vi "Flatten Pixmap 32-bit pixmap.vi"(4 "mask":u8[](array[numeric]), 5 "top left":cluster{"x":i16, "y":i16}, 6 "colors":u32[](array[numeric]), 7 "32-bit pixmap":u32[][](array[numeric]), 8 "1-bit pixmap":bool[][](array[boolean]), 9 "4-bit pixmap":u8[][](array[numeric]), 10 "8-bit pixmap":u8[][](array[numeric]), 11 "24-bit pixmap":u32[][](array[numeric])) -> (2 "image data":T1)   [LabVIEW 2021, in "Picture2D.lvlib"]
doc: "Converts pixmap data from a 2D array to a 1D array."
uses:
  Picture2D/Picture2D.lvlib
  <vilib>/picture/picture.llb/imagedata.ctl
panel:
  in  "image data":T1
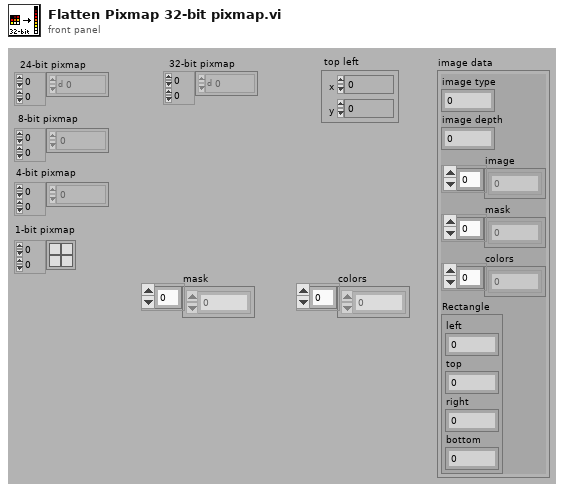
[diagram p1: front panel]
types:
  T1 = typedef "imagedata.ctl" = cluster{"image type":i32, "image depth":i32, "image":u8[], "mask":u8[], "colors":u32[], "Rectangle":cluster{"left":i16, "top":i16, "right":i16, "bottom":i16}}
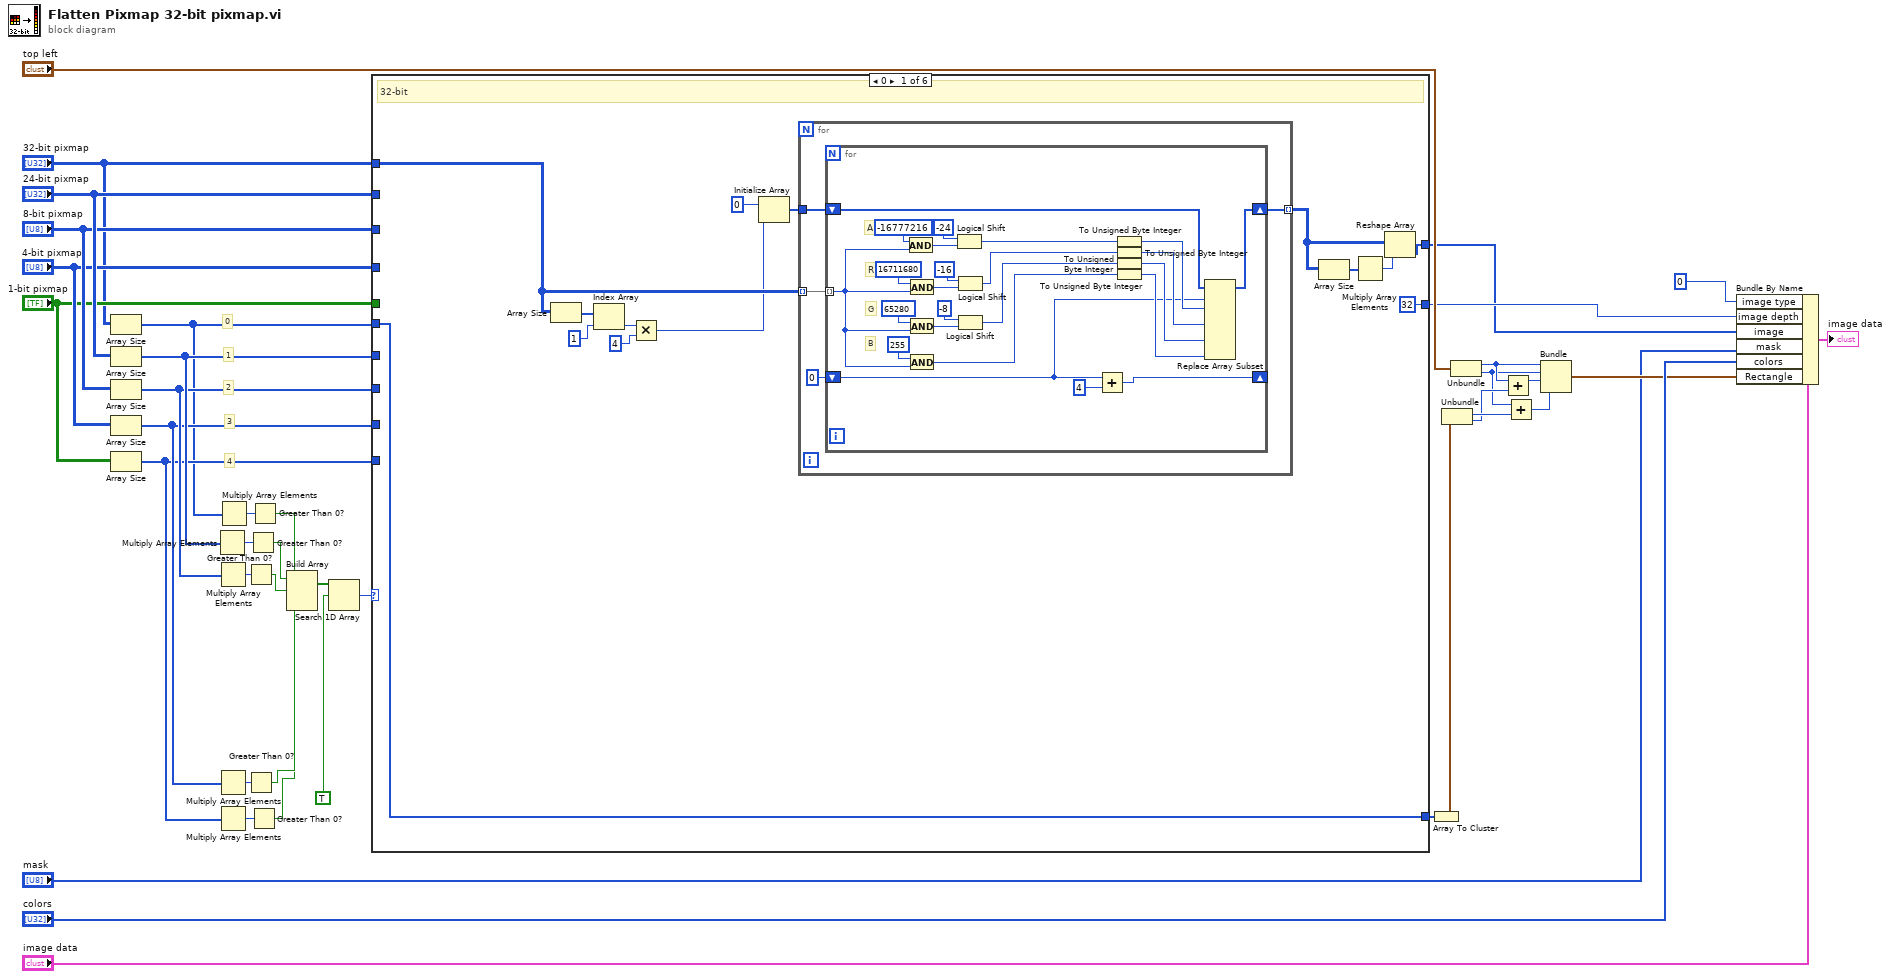
[diagram p0: block diagram]
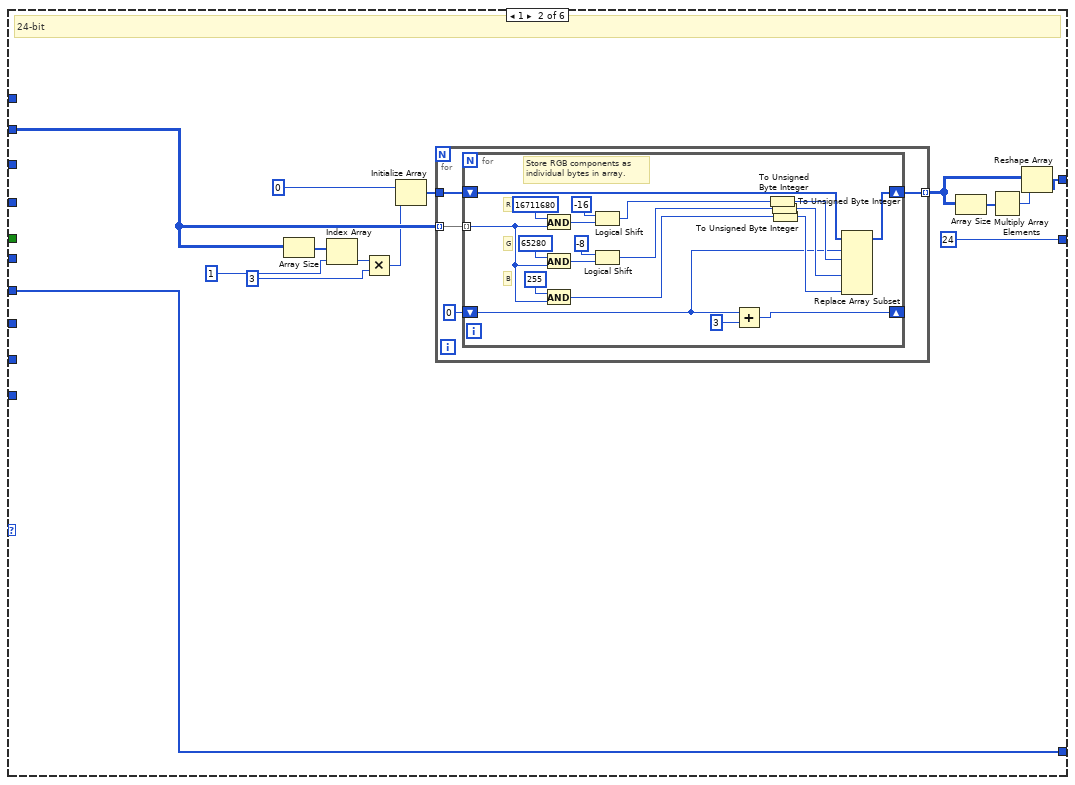
[diagram p2: hidden frame]
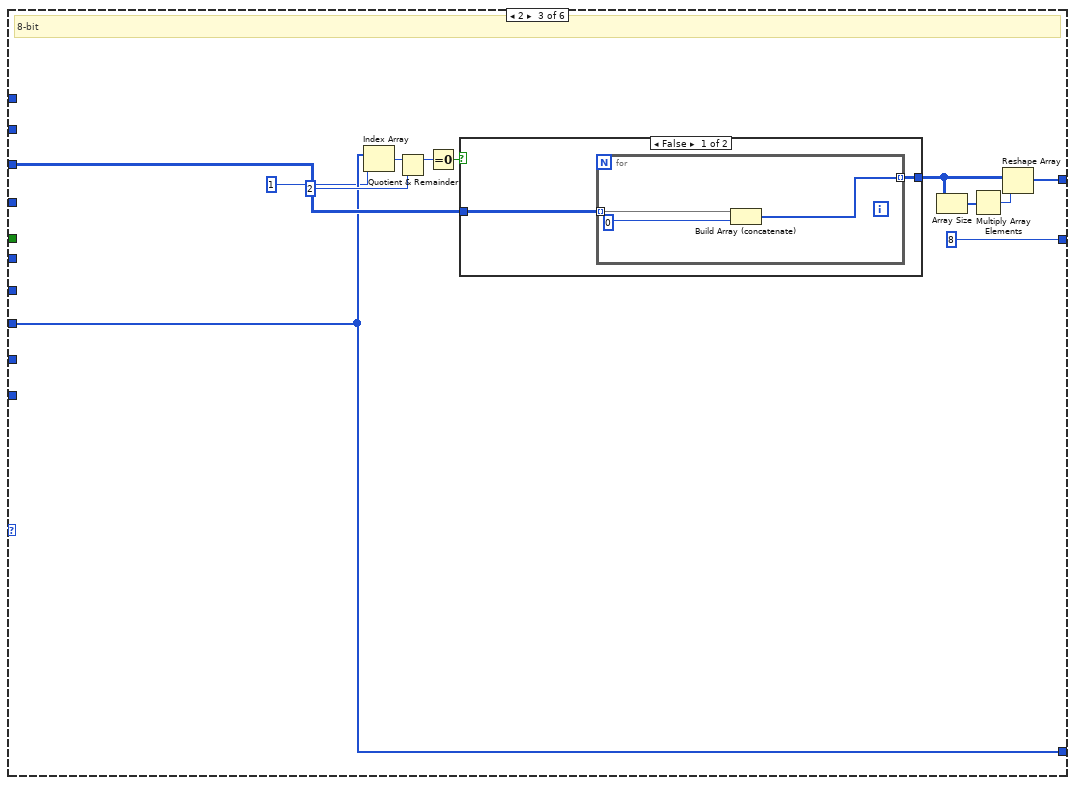
[diagram p3: hidden frame]
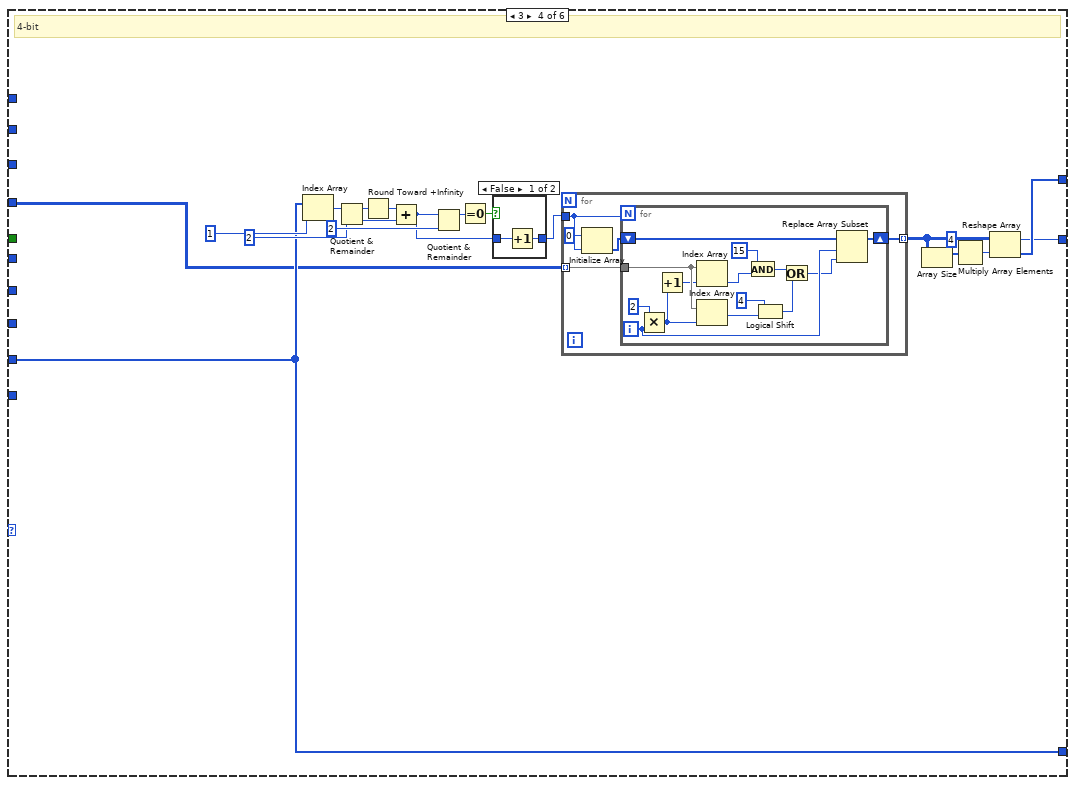
[diagram p5: hidden frame]
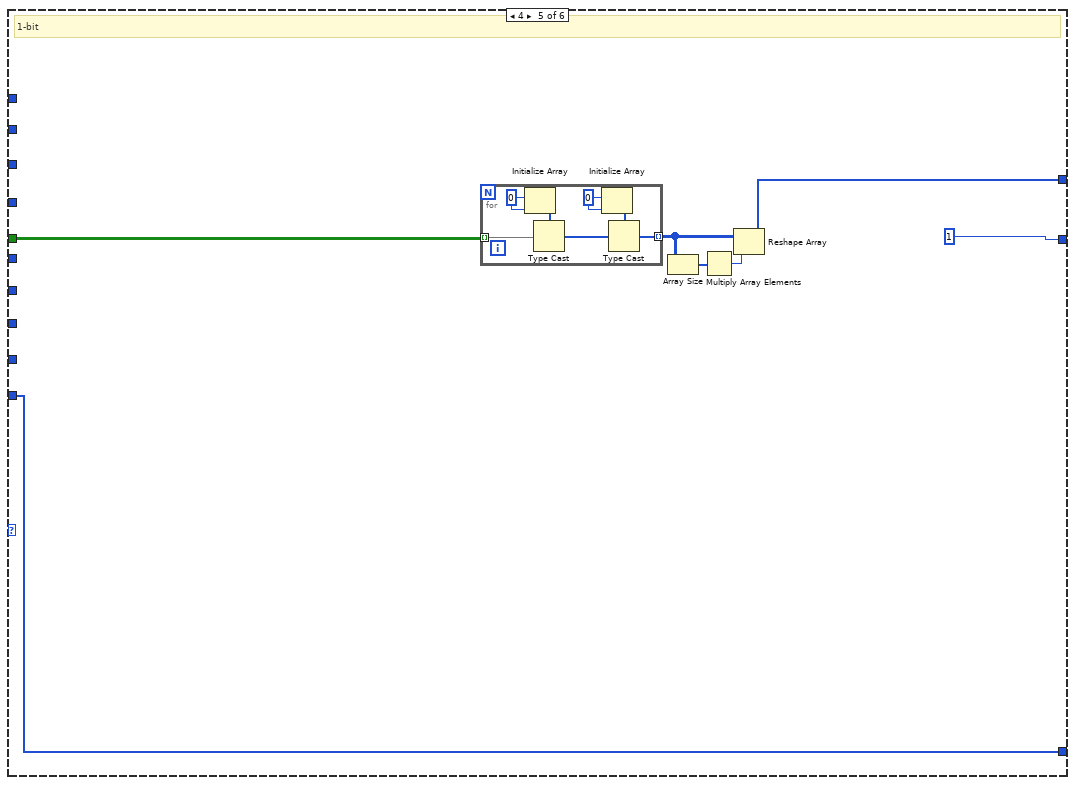
[diagram p7: hidden frame]
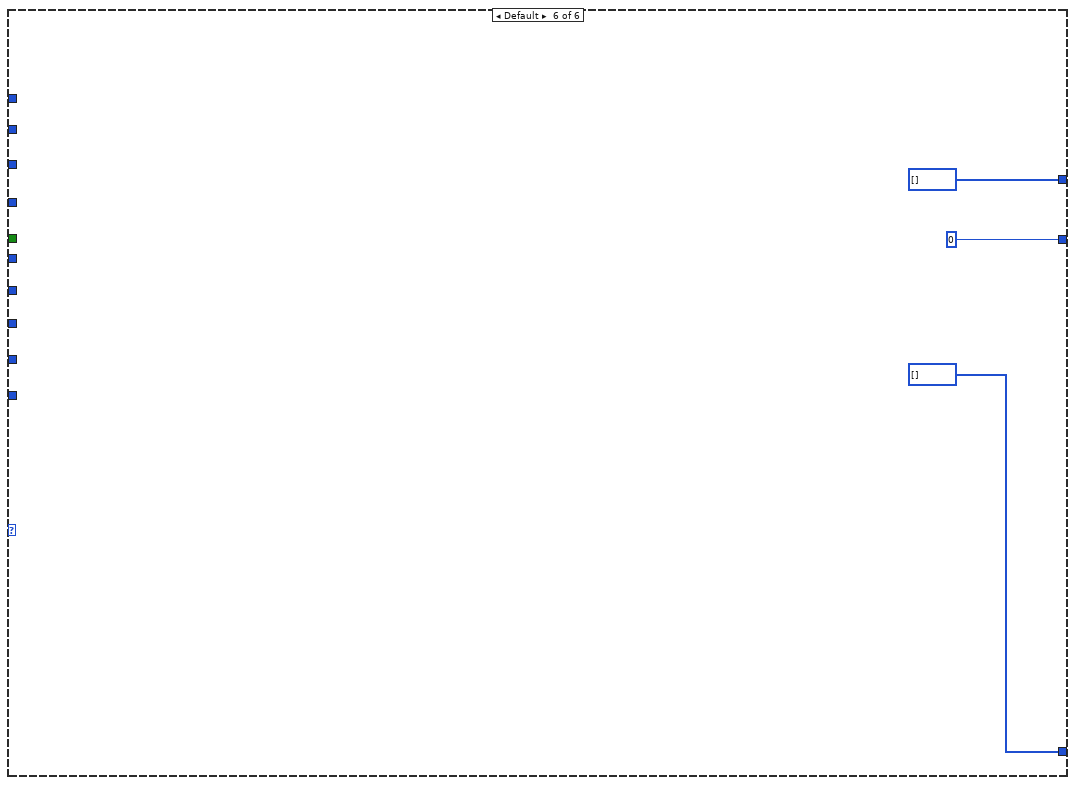
[diagram p8: hidden frame]
diagram:
  # "4"
  # "3"
  # "2"
  # "1"
  # "0"
  n1 = Array Size(array="32-bit pixmap") -> (size(s)=w1:i32[])
  n2 = Array Size(array="24-bit pixmap") -> (size(s)=w25:i32[])
  n3 = Array Size(array="8-bit pixmap") -> (size(s)=w24:i32[])
  n4 = Array Size(array="4-bit pixmap") -> (size(s)=w23:i32[])
  n5 = Array Size(array="1-bit pixmap") -> (size(s)=w22:i32[])
  n6 = Multiply Array Elements(1:w25) -> (0:w40:i32)
  n7 = Multiply Array Elements(1:w24) -> (0:w39:i32)
  n8 = Multiply Array Elements(1:w23) -> (0:w38:i32)
  n9 = Multiply Array Elements(1:w22) -> (0:w37:i32)
  n10 = Multiply Array Elements(1:w1) -> (0:w4:i32)
  n11 = Greater Than 0?(x=w39) -> (x > 0?=w34:bool)
  n12 = Greater Than 0?(x=w38) -> (x > 0?=w33:bool)
  n13 = Greater Than 0?(x=w40) -> (x > 0?=w35:bool)
  n14 = Greater Than 0?(x=w37) -> (x > 0?=w32:bool)
  n15 = Greater Than 0?(x=w4) -> (x > 0?=w2:bool)
  n16 = Build Array(w2, w35, w34, w33, w32) -> (w36:bool[])
  n17 = Search 1D Array(1D array=w36, element=TRUE) -> (index of element=w30:i32)  [unwired: 1 in]
  n18 = case shown="0" w30 {
    tunnel: [w54 w93 w126 w142 w180 u8[] [] ("8-bit pixmap")] -> w6
    tunnel: "24-bit pixmap" -> [_ w90 _ _ _ _]
    tunnel: "8-bit pixmap" -> [_ _ w125 _ _ _]
    tunnel: "4-bit pixmap" -> [_ _ _ w138 _ _]
    tunnel: "1-bit pixmap" -> [_ _ _ _ w181 _]
    tunnel: [32 24 8 4 1 0] -> w10
    tunnel: w25 -> [_ w91 _ _ _ _]
    tunnel: w24 -> [_ _ w122 _ _ _]
    tunnel: w23 -> [_ _ _ w140 _ _]
    tunnel: w22 -> [_ _ _ _ w178 _]
    tunnel: [w51 w91 w122 w140 w178 i32[] []] -> w21
    tunnel: "32-bit pixmap" -> [w52 _ _ _ _ _]
    tunnel: w1 -> [w51 _ _ _ _ _]
    frame 0 {
      # "32-bit"
      n19 = Array Size(array=w52) -> (size(s)=w47:i32[])
      n20 = Index Array(array=w47, index=1) -> (element=w45:i32)
      n21 = Multiply(x=w45, y=4) -> (x*y=w43:i32)
      n22 = Initialize Array(u8 0, w43) -> (w41:u8[])
      n23 = for {
        tunnel: w52 -> [w56] mode=indexing
        tunnel: [w58] -> w48 mode=indexing
        tunnel: w41 -> [w55]
        n24 = for {
          tunnel: w56 -> [w59] mode=indexing
          shift-right: [w67] -> w58
          shift-left: w55 -> [w68]
          shift-right: [w66] -> _
          shift-left: 0 -> [w60]
          # "A"
          # "B"
          # "G"
          # "R"
          n25 = And(x=-16777216, y=w59) -> (x .and. y?=w63:u32)
          n26 = And(x=16711680, y=w59) -> (x .and. y?=w77:u32)
          n27 = And(x=65280, y=w59) -> (x .and. y?=w76:u32)
          n28 = And(x=255, y=w59) -> (x .and. y?=w73:u32)
          n29 = Logical Shift(y=i8 -24, x=w63) -> (x << y=w62:u32)
          n30 = Logical Shift(y=i8 -16, x=w77) -> (x << y=w75:u32)
          n31 = Logical Shift(y=i8 -8, x=w76) -> (x << y=w74:u32)
          n32 = Add(x=w60, y=4) -> (x+y=w66:i32)
          n33 = To Unsigned Byte Integer(number=w62) -> (unsigned 8bit integer=w61:u8)
          n34 = To Unsigned Byte Integer(number=w75) -> (unsigned 8bit integer=w71:u8)
          n35 = To Unsigned Byte Integer(number=w74) -> (unsigned 8bit integer=w70:u8)
          n36 = To Unsigned Byte Integer(number=w73) -> (unsigned 8bit integer=w69:u8)
          n37 = Replace Array Subset(array=w68, new element #1=w61, index #1=w60, new element #2=w71, new element #3=w70, new element #4=w69) -> (w67:u8[])  [unwired: 3 in]
        }
      }
      n38 = Array Size(array=w48) -> (size(s)=w49:i32[])
      n39 = Multiply Array Elements(1:w49) -> (0:w50:i32)
      n40 = Reshape Array(w48, w50) -> (w54:u8[])
    }
    frame 1 {
      # "24-bit"
      n41 = Array Size(array=w90) -> (size(s)=w89:i32[])
      n42 = Index Array(array=w89, index=1) -> (element=w87:i32)
      n43 = Multiply(x=w87, y=3) -> (x*y=w85:i32)
      n44 = Initialize Array(u8 0, w85) -> (w83:u8[])
      n45 = for {
        tunnel: w90 -> [w98] mode=indexing
        tunnel: [w100] -> w94 mode=indexing
        tunnel: w83 -> [w97]
        n46 = for {
          tunnel: w98 -> [w109] mode=indexing
          shift-right: [w103] -> w100
          shift-left: w97 -> [w104]
          shift-right: [w102] -> _
          shift-left: 0 -> [w101]
          # "B"
          # "G"
          # "R"
          # "Store RGB components as\nindividual bytes in array."
          n47 = And(x=16711680, y=w109) -> (x .and. y?=w114:u32)
          n48 = And(x=65280, y=w109) -> (x .and. y?=w113:u32)
          n49 = And(x=255, y=w109) -> (x .and. y?=w110:u32)
          n50 = Logical Shift(y=i8 -16, x=w114) -> (x << y=w112:u32)
          n51 = Logical Shift(y=i8 -8, x=w113) -> (x << y=w111:u32)
          n52 = Add(x=w101, y=3) -> (x+y=w102:i32)
          n53 = To Unsigned Byte Integer(number=w112) -> (unsigned 8bit integer=w107:u8)
          n54 = To Unsigned Byte Integer(number=w111) -> (unsigned 8bit integer=w106:u8)
          n55 = To Unsigned Byte Integer(number=w110) -> (unsigned 8bit integer=w105:u8)
          n56 = Replace Array Subset(array=w104, new element #1=w107, index #1=w101, new element #2=w106, new element #3=w105) -> (w103:u8[])  [unwired: 2 in]
        }
      }
      n57 = Array Size(array=w94) -> (size(s)=w95:i32[])
      n58 = Multiply Array Elements(1:w95) -> (0:w96:i32)
      n59 = Reshape Array(w94, w96) -> (w93:u8[])
    }
    frame 2 {
      # "8-bit"
      n60 = Index Array(array=w122, index=1) -> (element=w121:i32)
      n61 = Quotient & Remainder(x=w121, y=2) -> (x-y*floor(x/y)=w127:i32)  [unwired: 1 out]
      n62 = Equal To 0?(x=w127) -> (x = 0?=w124:bool)
      n63 = case shown="False" w124 {
        tunnel: [w132 w137] -> w129
        tunnel: w125 -> [w133 w137]
        frame False {
          n64 = for {
            tunnel: w133 -> [w136] mode=indexing
            tunnel: [w134] -> w132 mode=indexing
            n65 = Build Array (concatenate)(w136, u8 0) -> (w134:u8[])
          }
        }
        frame True {
        }
      }
      n66 = Array Size(array=w129) -> (size(s)=w130:i32[])
      n67 = Multiply Array Elements(1:w130) -> (0:w131:i32)
      n68 = Reshape Array(w129, w131) -> (w126:u8[])
    }
    frame 3 {
      # "4-bit"
      n69 = Index Array(array=w140, index=1) -> (element=w154:i32)
      n70 = Quotient & Remainder(x=w154, y=2) -> (x-y*floor(x/y)=w148:i32, floor(x/y)=w146:i32)
      n71 = Round Toward +Infinity(x=w148) -> (ceil(x): smallest int >= x=w147:i32)
      n72 = Add(x=w147, y=w146) -> (x+y=w145:i32)
      n73 = Quotient & Remainder(x=w145, y=2) -> (x-y*floor(x/y)=w151:i32)  [unwired: 1 out]
      n74 = Equal To 0?(x=w151) -> (x = 0?=w150:bool)
      n75 = case shown="False" w150 {
        tunnel: w145 -> [w157 w158]
        tunnel: [w156 w158] -> w139
        frame False {
          n76 = Increment(x=w157) -> (x+1=w156:i32)
        }
        frame True {
        }
      }
      n77 = for {
        tunnel: w138 -> [w163] mode=indexing
        tunnel: [w162] -> w144 mode=indexing
        tunnel: w139 -> [w160]
        n78 = Initialize Array(u8 0, w160) -> (w159:u8[])
        n79 = for {
          N: w160 -> [_]
          tunnel: w163 -> [w177]
          shift-right: [w167] -> w162
          shift-left: w159 -> [w164]
          i -> [w166]
          n80 = Multiply(x=2, y=w166) -> (x*y=w175:i32)
          n81 = Increment(x=w175) -> (x+1=w174:i32)
          n82 = Index Array(array=w177, index=w174) -> (element=w173:u8)
          n83 = Index Array(array=w177, index=w175) -> (element=w171:u8)
          n84 = And(x=u8 15, y=w173) -> (x .and. y?=w170:u8)
          n85 = Logical Shift(y=u8 4, x=w171) -> (x << y=w169:u8)
          n86 = Or(x=w170, y=w169) -> (x .or. y?=w165:u8)
          n87 = Replace Array Subset(array=w164, new element=w165, index=w166) -> (w167:u8[])
        }
      }
      n88 = Array Size(array=w144) -> (size(s)=w143:i32[])
      n89 = Multiply Array Elements(1:w143) -> (0:w152:i32)
      n90 = Reshape Array(w144, w152) -> (w142:u8[])
    }
    frame 4 {
      # "1-bit"
      n91 = for {
        tunnel: [w188] -> w184 mode=indexing
        tunnel: w181 -> [w185] mode=indexing
        w187 = u8 0
        w190 = i16 0
        n92 = Initialize Array(w190, w190) -> (w191:i16[])
        n93 = Type Cast(type=w191, x=w185) -> (*(type *) &x=w189:i16[])
        n94 = Initialize Array(w187, w187) -> (w186:u8[])
        n95 = Type Cast(type=w186, x=w189) -> (*(type *) &x=w188:u8[])
      }
      n96 = Array Size(array=w184) -> (size(s)=w182:i32[])
      n97 = Multiply Array Elements(1:w182) -> (0:w183:i32)
      n98 = Reshape Array(w184, w183) -> (w180:u8[])
    }
    frame Default {
    }
  }
  n99 = Array To Cluster(array=w21) -> (cluster=w20:cluster{"[0]":i32, "[1]":i32})
  n100 = Unbundle(w20) -> ("[0]"=w19:i32, "[1]"=w16:i32)
  n101 = Unbundle("top left") -> ("x"=w17:i16, "y"=w15:i16)
  n102 = Add(x=w17, y=w16) -> (x+y=w13:i32)
  n103 = Add(x=w15, y=w19) -> (x+y=w14:i32)
  n104 = Bundle("x"=w17, "y"=w15, w13, w14) -> (w8:cluster{"x":i16, "y":i16, i32, i32})  [unwired: 1 in]
  n105 = Bundle By Name(cluster="image data", "image type"=u16 0, "image depth"=w10, "image"=w6, "mask"="mask", "colors"="colors", "Rectangle"=w8) -> (→"image data":T1)
